vi "Variaveis_Globais_para_Configurar_Aplicação_Paralelo.vi"() -> ()   [LabVIEW 2019]
panel:
  out "Configuração do Projeto":T1={"Application Name"="Novo", "Description"="Novo Projeto", "SPK-NC-CV-001"=FALSE, "SPK-NC-CV-002"=FALSE, "SPK-NC-CV-003"=FALSE, "SPK-NC-CV-004"=FALSE, "SPK-NO-CV-005"=FALSE, "SPK-NO-CV-006"=FALSE, "SPK-NO-CV-007"=FALSE, "SPK-NO-CV-008"=FALSE, "SPK-INV-001"=FALSE, "SPW-NC-CV-001"=FALSE, "SPW-NC-CV-002"=FALSE, "SPW-NC-CV-003"=FALSE, "SPW-NC-CV-004"=FALSE, "SPW-NO-CV-005"=FALSE, "SPW-NO-CV-006"=FALSE, "SPW-NO-CV-007"=FALSE, "SPW-NO-CV-008"=FALSE, "SPW-INV-001"=FALSE, "SKM-NC-CV-LAM"=FALSE, "SKM-NC-CV-COR"=FALSE, "SKM-FV-AR"=FALSE, "SKM-PV-TQ"=FALSE, "SKM-NC-CV-JMP"=FALSE, "SKM-FV-WF"=FALSE, "SKM-FV-KF"=FALSE, "SIW-NC-CV-001"=FALSE, "SIA-NC-CV-001"=FALSE, "SIK-NC-CV-001"=FALSE, "SIT-NC-CV-002"=FALSE, "SIT-NC-CV-001"=FALSE, "SIK-NC-CV-002"=FALSE, "SIW-NC-CV-002"=FALSE, "SKS-NC-CV-001"=FALSE, "SKS-NC-CV-002"=FALSE, "SKS-NC-CV-003"=FALSE, "Boolean"=FALSE, "Boolean 2"=FALSE, "SKS-NC-CV-006"=FALSE}
  # "SKID de Medição"
  # "SKID de BOMBAS"
  # "Querosene"
  # "Água"
  # "SKID de Separação"
  # "SKID de Injeção Trifásica"
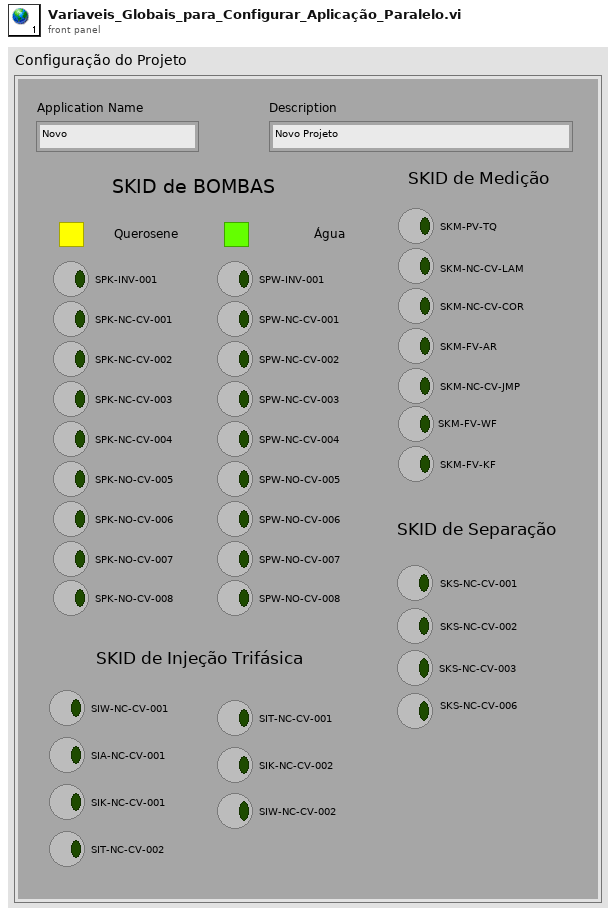
[diagram p1: front panel]
types:
  T1 = cluster{"Application Name":string, "Description":string, "SPK-NC-CV-001":bool, "SPK-NC-CV-002":bool, "SPK-NC-CV-003":bool, "SPK-NC-CV-004":bool, "SPK-NO-CV-005":bool, "SPK-NO-CV-006":bool, "SPK-NO-CV-007":bool, "SPK-NO-CV-008":bool, "SPK-INV-001":bool, "SPW-NC-CV-001":bool, "SPW-NC-CV-002":bool, "SPW-NC-CV-003":bool, "SPW-NC-CV-004":bool, "SPW-NO-CV-005":bool, "SPW-NO-CV-006":bool, "SPW-NO-CV-007":bool, "SPW-NO-CV-008":bool, "SPW-INV-001":bool, "SKM-NC-CV-LAM":bool, "SKM-NC-CV-COR":bool, "SKM-FV-AR":bool, "SKM-PV-TQ":bool, "SKM-NC-CV-JMP":bool, "SKM-FV-WF":bool, "SKM-FV-KF":bool, "SIW-NC-CV-001":bool, "SIA-NC-CV-001":bool, "SIK-NC-CV-001":bool, "SIT-NC-CV-002":bool, "SIT-NC-CV-001":bool, "SIK-NC-CV-002":bool, "SIW-NC-CV-002":bool, "SKS-NC-CV-001":bool, "SKS-NC-CV-002":bool, "SKS-NC-CV-003":bool, "Boolean":bool, "Boolean 2":bool, "SKS-NC-CV-006":bool}
diagram:
